vi "Fill Lists from DB (2nd Pass).vi"(4 "errorIN":errorcluster, 5 "colNames":string[](array[string]), 6 "lkupTableNames":string[](array[string]), 7 "RefNumArray":refnum<vi>[](array[refnum])) -> (0 "error OUT":errorcluster)   [LabVIEW 2015]
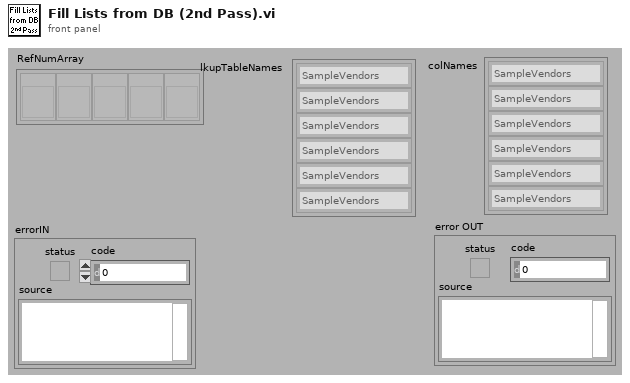
[diagram p1: front panel]
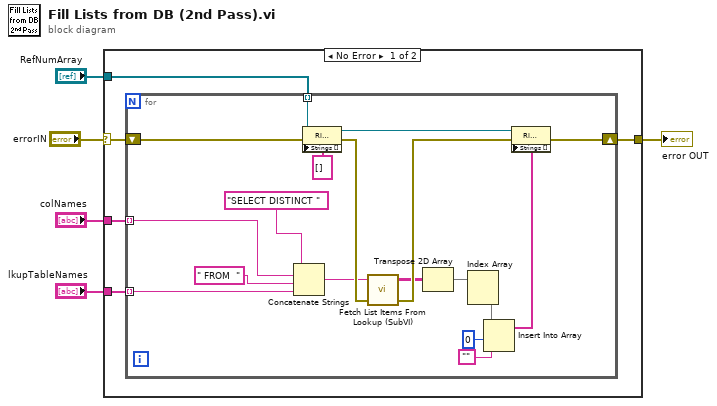
[diagram p0: block diagram]
diagram:
  n1 = case shown="No Error" "errorIN" {
    selector: "errorIN" -> [w9 w29]
    tunnel: [w10 w29] -> w5
    tunnel: "RefNumArray" -> [w8 _]
    tunnel: "lkupTableNames" -> [w7 _]
    tunnel: "colNames" -> [w6 _]
    frame No Error {
      n2 = for {
        tunnel: w8 -> [w19] mode=indexing
        tunnel: w7 -> [w14] mode=indexing
        shift-right: [w27] -> w10
        shift-left: w9 -> [w16]
        tunnel: w6 -> [w11] mode=indexing
        n3 = Concatenate Strings("SELECT DISTINCT " ("string"), w11, " FROM  " ("string"), w14) -> (w13:string)
        n4 = property class="Ring (strict)"(reference=w19, error in=w16, "Strings []"=string[] []) -> (reference out=w18:refnum<vi>, error out=w17:errorcluster)
        n5 = call "Fetch List Items From Lookup (SubVI).vi"("error IN"=w17, "Query"=w13) -> ("error OUT"=w28:errorcluster, "recordset data"=w22:string[][])  [unwired: 2 out]
        n6 = Transpose 2D Array(2D array=w22) -> (transposed array=w23:string[][])
        n7 = Index Array(array=w23) -> (element=w26:string[])  [unwired: 2 in]
        n8 = Insert Into Array "Insert Into Array"(array=w26, index=0, new element="" ("new element/subarray")) -> (w21:string[])
        n9 = property class="Ring (strict)"(reference=w18, error in=w28, "Strings []"=w21) -> (error out=w27:errorcluster)  [unwired: 1 out]
      }
    }
    frame Error {
    }
  }
  "error OUT" <- w5
